vi "globalSetUp.vi"(8 "error in":errorcluster, 11 "Deployment in":refnum<class "AIM Deployment.lvclass">) -> (0 "error out":errorcluster, 3 "Deployment out":refnum<class "AIM Deployment.lvclass">)   [LabVIEW 2020, in "AIM Deployment.lvclass"]
uses:
  AIM Deployment.lvclass
  <vilib>/NI/VeriStand Custom Device Testing Tools/VeriStandTestUtilities/VeriStandTestUtilities.lvlib
  Scripting/AIM/AIM ARINC 429 Scripting.lvlib
  Shared/Device Parameters.ctl
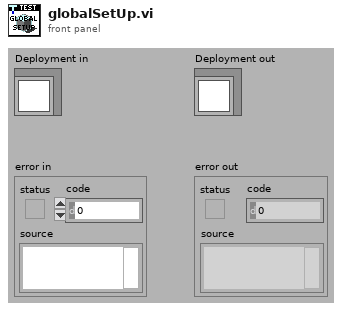
[diagram p1: front panel]
types:
  T1 = typedef "Device Parameters.ctl" = cluster{"pxi slot":u8}
  T2 = typedef "Custom Device API.lvlib/Custom Device Item Ref.ctl" = u64
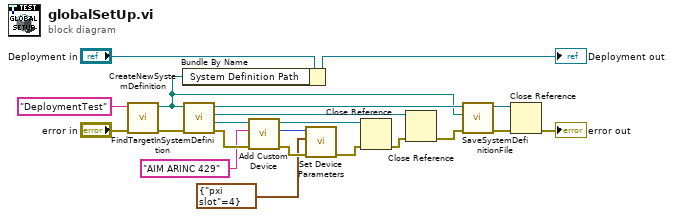
[diagram p0: block diagram]
diagram:
  n1 = call <vilib>:"CreateNewSystemDefinition.vi"("error in"="error in", "System Definition Name"="DeploymentTest") -> ("error out"=w13:errorcluster, "System Definition Path"=w14:path)  [unwired: 8 in]
  n2 = Bundle By Name(cluster="Deployment in", "System Definition Path"=w14) -> (→"Deployment out":refnum<class "AIM Deployment.lvclass">)
  n3 = call <vilib>:"FindTargetInSystemDefinition.vi"("error in"=w13, "system definition path"=w14) -> ("error out"=w7:errorcluster, "Target"=w8:refnum<k24>, "Root"=w20:refnum<k24>, "System Definition"=w21:refnum<k24>)  [unwired: 6 in]
  n4 = call "Add Custom Device.vi"("error in"=w7, "name"="AIM ARINC 429", "target"=w8) -> ("error out"=w4:errorcluster, "AIM ARINC 429 custom device"=w5:T2, "target out"=w2:refnum<k24>)  [unwired: 6 in]
  n5 = call "Set Device Parameters.vi"("error in"=w4, "device parameters"=T1 {"pxi slot"=4}, "custom device"=w5) -> ("error out"=w3:errorcluster)  [unwired: 7 in, 1 out]
  n6 = Close Reference(reference=w2, error in (no error)=w3) -> (error out=w18:errorcluster)
  n7 = Close Reference(reference=w20, error in (no error)=w18) -> (error out=w19:errorcluster)
  n8 = call <vilib>:"SaveSystemDefinitionFile.vi"("error in (no error)"=w19, "System Definition File in"=w14, "System Definition Reference in"=w21) -> ("error out"=w17:errorcluster, "System Definition Reference out"=w16:refnum<k24>)  [unwired: 7 in]
  n9 = Close Reference(reference=w16, error in (no error)=w17) -> (error out=→"error out":errorcluster)
